vi "flow meter test.vi"() -> ()   [LabVIEW 2019]
uses:
  <vilib>/eio/EIONode/EIONode.xnode
  <vilib>/Platform/TimedLoop/XDataNode/XDataNode.xnode
  <vilib>/Platform/TimedLoop/XDataNode/nitl_modes.ctl
  <vilib>/Platform/TimedLoop/XDataNode/XDNodeRunTimeDep.lvlib
  <vilib>/Platform/TimedLoop/XDataNode/wakeup.ctl
  <vilib>/Platform/TimedLoop/XDataNode/timing_clust.ctl
  <vilib>/rvi/eio/common/nirviEmuTemplateMethod_errors.vi
panel:
  out "Period 6":u32
  out "Period 5":u32
  out "Period 4":u32
  out "Period 3":u32
  out "Period 2":u32
  out "Period 1":u32
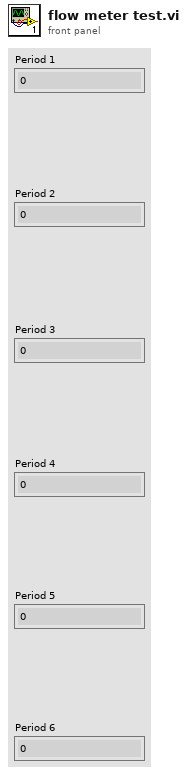
[diagram p1: front panel]
types:
  T1 = typedef "XDNodeRunTimeDep.lvlib/timing_clust.ctl" = cluster{"Expected End [f-1]":u64, "Actual End [f-1]":u64, "Finished Late? [f-1]":bool, "Expected End [i-1]":u64, "Actual End [i-1]":u64, "Finished Late? [i-1]":bool, "Expected Start [i]":u64, "Actual Start [i]":u64, "Expected Start [f]":u64, "Actual Start [f]":u64, "Source Name":string, "Structure Name":string, "Period":i64, "Deadline":i64, "Offset":i64, "Start":i64, "Priority":i32, "Timeout":i32, "Mode":T2, "Wakeup Reason":T3, "Error":errorcluster, "Source Type":string, "Secondary Source Type":string, "Global End Time":u64, "Global Start Time":u64, "Frame Duration":u64, "Iteration Duration":u64, "Assigned CPU":i32, "I/O Scan Engine Mode":u32}
  T2 = typedef "XDNodeRunTimeDep.lvlib/nitl_modes.ctl" = enum32{"No Change", "Process missed periods, maintain original phase", "Discard missed periods, maintain original phase", "Process missed periods, ignore original phase", "Discard missed periods, ignore original phase"}
  T3 = typedef "XDNodeRunTimeDep.lvlib/wakeup.ctl" = enum32{"Normal", "Aborted", "Asynchronous wakeup", "Timing source error", "Timed loop error", "Timeout"}
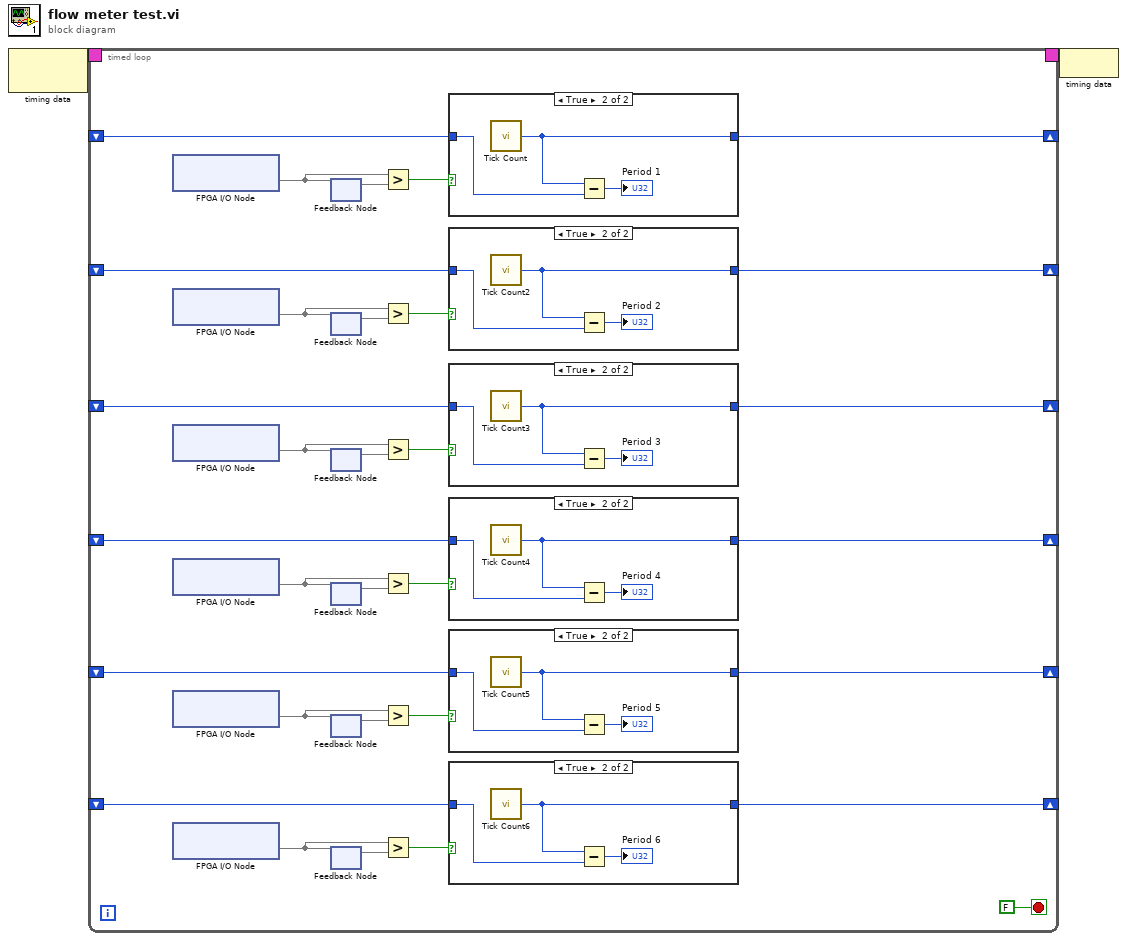
[diagram p0: block diagram]
diagram:
  n1 = node-c288() -> (w2:T1)  [unwired: 1 in]
  n2 = timed-loop {
    timing: w2 -> [_]
    timing-out: [_] -> w1
    shift-right: [w29] -> _
    shift-left: _ -> [w28]
    shift-right: [w26] -> _
    shift-left: _ -> [w27]
    shift-right: [w19] -> _
    shift-left: _ -> [w18]
    shift-right: [w16] -> _
    shift-left: _ -> [w17]
    shift-right: [w9] -> _
    shift-left: _ -> [w8]
    shift-right: [w6] -> _
    shift-left: _ -> [w7]
    stop <- FALSE stop-if-true
    n3 = xnode "FPGA I/O Node"() -> ("RMC/DIO32"=w32)  [unwired: 1 in, 1 out]
    n4 = xnode "FPGA I/O Node"() -> ("RMC/DIO33"=w23)  [unwired: 1 in, 1 out]
    n5 = xnode "FPGA I/O Node"() -> ("RMC/DIO34"=w22)  [unwired: 1 in, 1 out]
    n6 = xnode "FPGA I/O Node"() -> ("RMC/DIO35"=w13)  [unwired: 1 in, 1 out]
    n7 = xnode "FPGA I/O Node"() -> ("RMC/DIO36"=w12)  [unwired: 1 in, 1 out]
    n8 = xnode "FPGA I/O Node"() -> ("RMC/DIO37"=w3)  [unwired: 1 in, 1 out]
    n9 = feedback-in #1(w32) -> ()
    n10 = feedback #1() -> (w31)  [unwired: 1 in]
    n11 = feedback #2() -> (w24)  [unwired: 1 in]
    n12 = feedback-in #2(w23) -> ()
    n13 = feedback #3() -> (w21)  [unwired: 1 in]
    n14 = feedback-in #3(w22) -> ()
    n15 = feedback #4() -> (w14)  [unwired: 1 in]
    n16 = feedback-in #4(w13) -> ()
    n17 = feedback #5() -> (w11)  [unwired: 1 in]
    n18 = feedback-in #5(w12) -> ()
    n19 = feedback #6() -> (w4)  [unwired: 1 in]
    n20 = feedback-in #6(w3) -> ()
    n21 = Greater?(x=w32, y=w31) -> (0:w30:bool)
    n22 = Greater?(x=w23, y=w24) -> (0:w25:bool)
    n23 = Greater?(x=w22, y=w21) -> (0:w20:bool)
    n24 = Greater?(x=w13, y=w14) -> (0:w15:bool)
    n25 = Greater?(x=w12, y=w11) -> (0:w10:bool)
    n26 = Greater?(x=w3, y=w4) -> (0:w5:bool)
    n27 = case shown="True" w30 {
      tunnel: [w54 w56] -> w29
      tunnel: w28 -> [w54 w55]
      frame False {
      }
      frame True {
        n28 = call "Tick Count"() -> ("Tick Count(uSec)"=w56:u32)
        n29 = Subtract(x=w56, y=w55) -> (x-y=→"Period 1":u32)
      }
    }
    n30 = case shown="True" w25 {
      tunnel: [w50 w52] -> w26
      tunnel: w27 -> [w50 w51]
      frame False {
      }
      frame True {
        n31 = call "Tick Count2"() -> ("Tick Count(uSec)"=w52:u32)
        n32 = Subtract(x=w52, y=w51) -> (x-y=→"Period 2":u32)
      }
    }
    n33 = case shown="True" w20 {
      tunnel: [w46 w48] -> w19
      tunnel: w18 -> [w46 w47]
      frame False {
      }
      frame True {
        n34 = call "Tick Count3"() -> ("Tick Count(uSec)"=w48:u32)
        n35 = Subtract(x=w48, y=w47) -> (x-y=→"Period 3":u32)
      }
    }
    n36 = case shown="True" w15 {
      tunnel: [w42 w44] -> w16
      tunnel: w17 -> [w42 w43]
      frame False {
      }
      frame True {
        n37 = call "Tick Count4"() -> ("Tick Count(uSec)"=w44:u32)
        n38 = Subtract(x=w44, y=w43) -> (x-y=→"Period 4":u32)
      }
    }
    n39 = case shown="True" w10 {
      tunnel: [w38 w40] -> w9
      tunnel: w8 -> [w38 w39]
      frame False {
      }
      frame True {
        n40 = call "Tick Count5"() -> ("Tick Count(uSec)"=w40:u32)
        n41 = Subtract(x=w40, y=w39) -> (x-y=→"Period 5":u32)
      }
    }
    n42 = case shown="True" w5 {
      tunnel: [w34 w36] -> w6
      tunnel: w7 -> [w34 w35]
      frame False {
      }
      frame True {
        n43 = call "Tick Count6"() -> ("Tick Count(uSec)"=w36:u32)
        n44 = Subtract(x=w36, y=w35) -> (x-y=→"Period 6":u32)
      }
    }
  }
  n45 = node-c288(w1) -> ()
